vi "XIPIN_LTE_RACH_Detector_2_0.vi"   [LabVIEW 2017]
doc: "The Xilinx LTE RACH Detector LogiCORE performs receiver correlation against P-RACH data encoded according to the 3GPP TS 36.211 v9.0 (2009-12) \"Physical Channels and Modulation\" specification. This correlation result can be used to determine RACH timing for an LTE Uplink Reciever.\n------------------------------------\n<b>Need License</b> : Yes"
uses:
  <vilib>/rvi/XilinxIP/XIPIN_XNode/niFpgaXIPIN.xnode
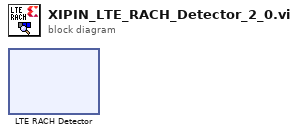
[diagram p0: block diagram]
diagram:
  n1 = xnode ("LTE RACH Detector")() -> ()
